vi "Timing-Measure Precision.vi"() -> ()   [LabVIEW 2020]
uses:
  <vilib>/Analysis/polynomials.llb/Unique Numbers and Multiplicity (DBL).vi
  <vilib>/Analysis/NI_AALPro.lvlib
panel:
  out "Precision (ms)":dbl
  out "Num unique":i32
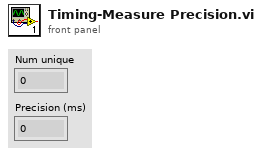
[diagram p1: front panel]
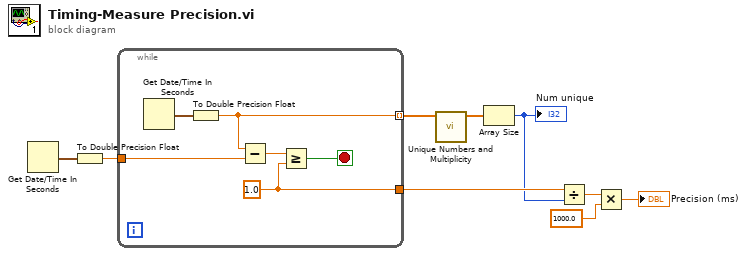
[diagram p0: block diagram]
diagram:
  n1 = Get Date/Time In Seconds() -> (seconds since 1Jan1904=w9:timestamp)
  n2 = To Double Precision Float(number=w9) -> (double precision float=w8:dbl)
  n3 = while {
    tunnel: w8 -> [w13]
    tunnel: [w14] -> w7 mode=indexing
    tunnel: [w10] -> w5
    stop <- w11 stop-if-true
    w10 = 1.0 ("y")
    n4 = Get Date/Time In Seconds() -> (seconds since 1Jan1904=w15:timestamp)
    n5 = To Double Precision Float(number=w15) -> (double precision float=w14:dbl)
    n6 = Subtract(x=w14, y=w13) -> (x-y=w12:dbl)
    n7 = Greater Or Equal?(x=w12, y=w10) -> (x >= y?=w11:bool)
  }
  n8 = call-poly <vilib>:"Unique Numbers and Multiplicity.vi"("Numbers"=w7) -> ("Unique Numbers"=w6:dbl[])  [unwired: 8 in, 2 out]
  n9 = Array Size(array=w6) -> (size(s)=w4:i32)
  "Num unique" <- w4
  n10 = Divide(x=w5, y=w4) -> (x/y=w3:dbl)
  n11 = Multiply(x=w3, y=1000.0) -> (x*y=→"Precision (ms)":dbl)
